vi "Handle Error.vi"(7 "Mode":T1(ring), 8 "error in (no error)":errorcluster, 9 "Test Method Name":string, 11 "Test Case Result In":T2) -> (0 "error out":errorcluster, 3 "Test Case Result Out":T2)   [LabVIEW 2020, in "Test Case Result.lvlib"]
uses:
  Test Case Result.lvlib
  Test Case Result.ctl
  Method Result/Method Result.ctl
  Assertion Result/Public/TypeDefs/Status.ctl
  Assertion Result/Assertion Result.ctl
  Assertion Result/Public/TypeDefs/Assertion Type.ctl
  <vilib>/Utility/miscctls.llb/LVMapReplaceAction.ctl
  Method Result/Method Result.lvlib
  Assertion Result/Assertion Result.lvlib
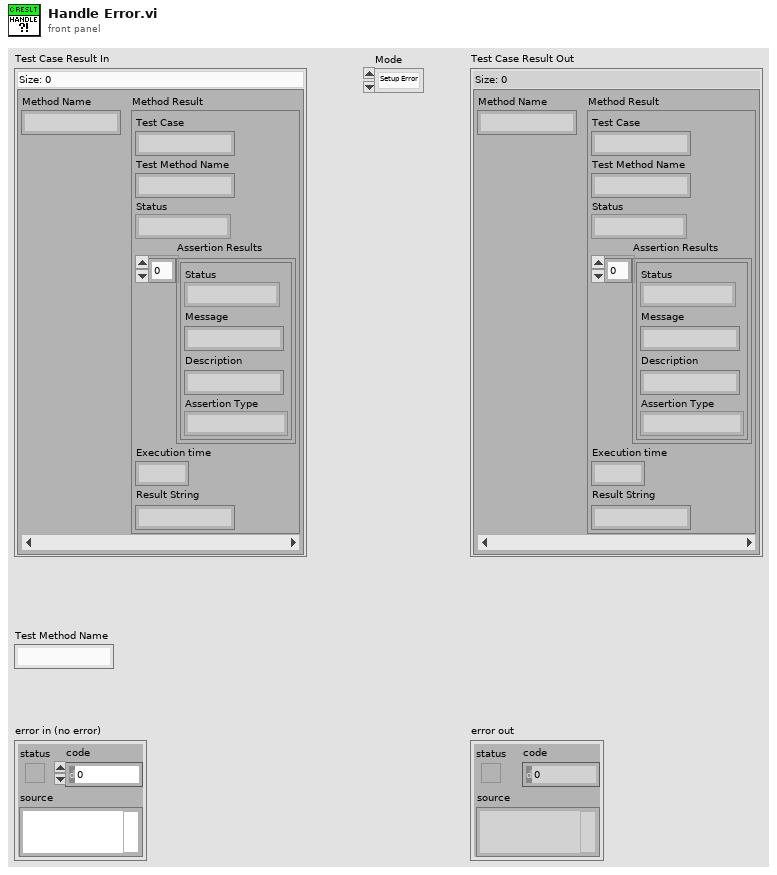
[diagram p1: front panel]
types:
  T1 = enum16{"Setup Error", "Teardown Error", "Broken", "Test Method Error"}
  T2 = typedef "Test Case Result.lvlib/Test Case Result.ctl" = map{string, T3}
  T3 = typedef "Method Result.lvlib/Method Result.ctl" = cluster{"Test Case":string, "Test Method Name":string, "Status":T4, "Assertion Results":T5[], "Execution time":dbl, "Result String":string}
  T4 = typedef "Assertion Result.lvlib/Status.ctl" = enum16{"Pass", "Fail", "Error", "Skipped", "Setup Error", "Broken", "Teardown Error"}
  T5 = typedef "Assertion Result.lvlib/Assertion Result.ctl" = cluster{"Status":T4, "Message":string, "Description":string, "Assertion Type":T6}
  T6 = typedef "Assertion Result.lvlib/Assertion Type.ctl" = enum16{"None", "Pass", "Fail", "Skip", "Pass if Equal", "Fail if Equal", "Pass if Error", "Fail if Error", "Pass if", "Fail if"}
  T7 = typedef "LVMapReplaceAction.ctl" = enum32{"Modify Entry only if found", "Add or Modify Entry", "Delete Entry"}
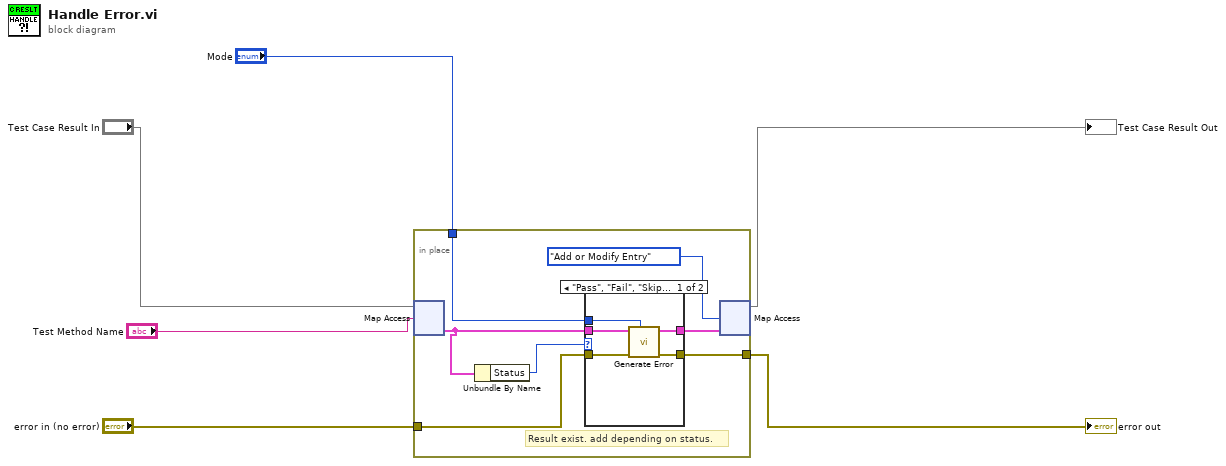
[diagram p0: block diagram]
diagram:
  n1 = in-place {
    in-place-border: "Mode" -> [w12]
    in-place-border: "error in (no error)" -> [w10]
    in-place-border: [w11] -> w4
    # "Result exist. add depending on status."
    n2 = in-place-map #1("Test Case Result In", "Test Method Name") -> (w7:T3)  [unwired: 1 in, 1 out]
    n3 = Unbundle By Name(w7) -> ("Status"=w8:T4)
    n4 = case shown="\"Pass\", \"Fail\", \"Skipped\"" w8 {
      tunnel: w7 -> [w18 w20]
      tunnel: [w17 w20] -> w13
      tunnel: w10 -> [w16 w19]
      tunnel: [w15 w19] -> w11
      tunnel: w12 -> [w14 _]
      frame "Pass", "Fail", "Skipped" {
        n5 = call "Generate Error.vi"("Mode"=w14, "error in (no error)"=w16, "Method Result In"=w18) -> ("error out"=w15:errorcluster, "Method Result Out"=w17:T3)  [unwired: 7 in]
      }
      frame Default {
      }
    }
    n6 = in-place-map #1(w13, LVMapReplaceAction."Add or Modify Entry" ("action")) -> (→"Test Case Result Out":T2)  [unwired: 2 out]
  }
  "error out" <- w4
